vi "ex13.vi"() -> ()   [LabVIEW 2019]
panel:
  in  "y 2":i32
  out "x+y":dbl
  in  "y":dbl
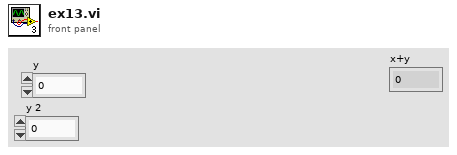
[diagram p1: front panel]
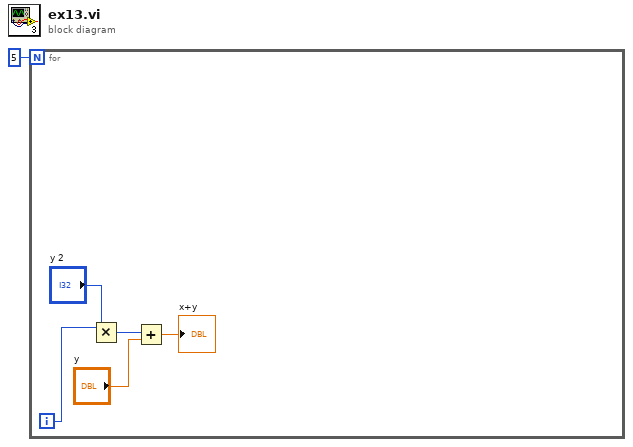
[diagram p0: block diagram]
diagram:
  n1 = for {
    N: 5 -> [_]
    i -> [w4]
    n2 = Multiply(x=w4, y="y 2") -> (x*y=w3:i32)
    n3 = Add(x=w3, y="y") -> (x+y=→"x+y":dbl)
  }
